vi "Init.vi"(8 "error in (no error)":errorcluster, 10 "Left Motor ID":u8, 11 "Right Motor ID":u8) -> (0 "error out":errorcluster)   [LabVIEW 2017, in "Drive Train.lvlib"]
uses:
  Drive Train.lvlib
  Controls/Library Information.ctl
  Controls/FGV Actions.ctl
  Controls/Motion Magic Parameters.ctl
  <vilib>/Rock Robotics/WPI/ThirdParty/Phoenix-LabVIEW/Motor Controller/Controls/CTRE_Phoenix_MotorControl_ControlMode.ctl
  Controls/Motor Controllers Parameters.ctl
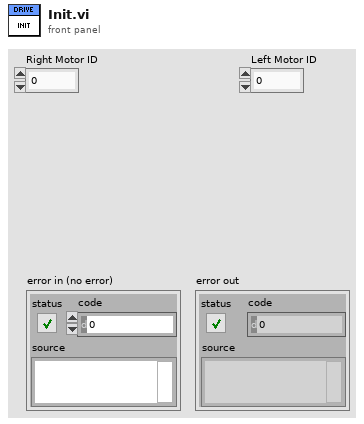
[diagram p1: front panel]
types:
  T1 = typedef "Drive Train.lvlib/Motor Controllers Parameters.ctl" = cluster{"Max Current (amps)":i32, "PID Buckets":cluster{"High Gear":i32, "High Gear Ramp":i32, "Low Gear":i32, "Low Gear Ramp":i32}}
  T2 = typedef "Drive Train.lvlib/Motion Magic Parameters.ctl" = cluster{"Native Units":dbl}
  T3 = typedef "Drive Train.lvlib/FGV Actions.ctl" = enum16{"Get", "Set"}
  T4 = typedef "Drive Train.lvlib/Library Information.ctl" = cluster{"Right Motor Name":string, "Left Motor Name":string, "Current Control Mode":T5, "Motion Magic Parameters":T2, "Motor Controllers Parameters":T1}
  T5 = typedef "CTRE_Phoenix_MotorControl_ControlMode.ctl" = u16
  T6 = typedef "WPI_MotorControlDeviceRef.ctl" = cluster{"DeviceStatus":errorcluster, "Type":T7, "PWM":cluster{"PWM Channel":T8, "DeadBand":T9}, "CAN":cluster{"Device Number":u8, "SetOutput VI Ref":variant, "GetOutput VI Ref":variant, "Enable VI Ref":variant, "Disable VI Ref":variant, "Data":variant}, "Invert":bool, "DIO PWM":cluster{"PWM \"Enable\" Channel":T8, "DIOChannel":T10, "PWM Rate":dbl}}
  T7 = typedef "WPI_MotorControlType.ctl" = enum16{"PWM", "CAN", "DIO PWM"}
  T8 = typedef "FPGA_DIOPWMChannel.ctl" = enum8{"PWM 0", "PWM 1", "PWM 2", "PWM 3", "PWM 4", "PWM 5", "PWM 6", "PWM 7", "PWM 8", "PWM 9", "PWM MXP 0", "PWM MXP 1", "PWM MXP 2", "PWM MXP 3", "PWM MXP 4", "PWM MXP 5", "PWM MXP 6", "PWM MXP 7", "PWM MXP 8", "PWM MXP 9", "Invalid"}
  T9 = typedef "WPI_PWMDeadband.ctl" = cluster{"Name":string, "maxPositivePwm":i32, "minPositivePwm":i32, "centerPwm":i32, "maxNegativePwm":i32, "minNegativePwm":i32, "angularRange":u16}
  T10 = typedef "FPGA_DIOChannel.ctl" = enum8{"DIO 0", "DIO 1", "DIO 2", "DIO 3", "DIO 4", "DIO 5", "DIO 6", "DIO 7", "DIO 8", "DIO 9", "DIO MXP 0", "DIO MXP 1", "DIO MXP 2", "DIO MXP 3", "DIO MXP 4", "DIO MXP 5", "DIO MXP 6", "DIO MXP 7", "DIO MXP 8", "DIO MXP 9", "DIO MXP 10", "DIO MXP 11", "DIO MXP 12", "DIO MXP 13", "DIO MXP 14", "DIO MXP 15", "SPI Port CS1", "SPI Port CS2", "SPI Port CS3", "SPI Port MISO", "SPI Port MOSI", "Invalid"}
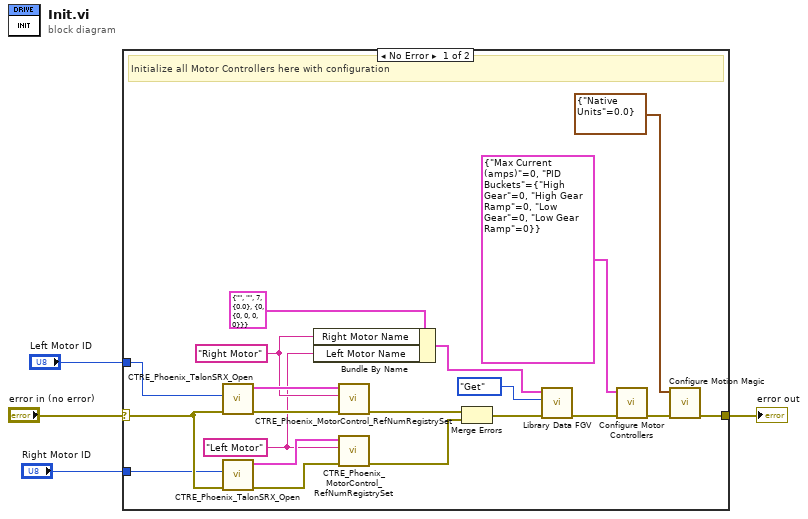
[diagram p0: block diagram]
diagram:
  n1 = case shown="No Error" "error in (no error)" {
    selector: "error in (no error)" -> [w20 w25]
    tunnel: [w8 w25] -> w3
    tunnel: "Left Motor ID" -> [w17 _]
    tunnel: "Right Motor ID" -> [w16 _]
    frame No Error {
      w10 = "Right Motor" ("refnum name")
      w9 = "Left Motor" ("refnum name")
      # "Initialize all Motor Controllers here with configuration"
      n2 = call <vilib>:"CTRE_Phoenix_TalonSRX_Open.vi"("error in"=w20, "Device Number"=w17) -> ("error out"=w24:errorcluster, "CAN Talon SRX Ref"=w23:T6)  [unwired: 8 in]
      n3 = call <vilib>:"CTRE_Phoenix_TalonSRX_Open.vi"("error in"=w20, "Device Number"=w16) -> ("error out"=w21:errorcluster, "CAN Talon SRX Ref"=w22:T6)  [unwired: 8 in]
      n4 = Bundle By Name(cluster=T4 {"Right Motor Name"="", "Left Motor Name"="", "Current Control Mode"=7, "Motion Magic Parameters"={"Native Units"=0.0}, "Motor Controllers Parameters"={"Max Current (amps)"=0, "PID Buckets"={"High Gear"=0, "High Gear Ramp"=0, "Low Gear"=0, "Low Gear Ramp"=0}}} ("Library Information in"), "Right Motor Name"=w10, "Left Motor Name"=w9) -> (w11:T4)
      n5 = call <vilib>:"CTRE_Phoenix_MotorControl_RefNumRegistrySet.vi"("error in (no error)"=w24, "refnum name"=w10, "PhoenixMotorControlDevRef"=w23) -> ("error out"=w18:errorcluster)  [unwired: 7 in, 1 out]
      n6 = call <vilib>:"CTRE_Phoenix_MotorControl_RefNumRegistrySet.vi"("error in (no error)"=w21, "refnum name"=w9, "PhoenixMotorControlDevRef"=w22) -> ("error out"=w19:errorcluster)  [unwired: 7 in, 1 out]
      n7 = Merge Errors(w18, w19) -> (w15:errorcluster)
      n8 = call "Library Data FGV.vi"("error in (no error)"=w15, "FGV Actions"=FGV_Actions."Get", "Library Information in"=w11) -> ("error out"=w14:errorcluster)  [unwired: 7 in, 1 out]
      n9 = call "Configure Motor Controllers.vi"("error in (no error)"=w14, "Motion Magic Parameters"=T1 {"Max Current (amps)"=0, "PID Buckets"={"High Gear"=0, "High Gear Ramp"=0, "Low Gear"=0, "Low Gear Ramp"=0}}) -> ("error out"=w6:errorcluster)  [unwired: 9 in]
      n10 = call "Configure Motion Magic.vi"("error in (no error)"=w6, "Motion Magic Parameters"=T2 {"Native Units"=0.0}) -> ("error out"=w8:errorcluster)  [unwired: 9 in]
    }
    frame Error {
    }
  }
  "error out" <- w3
